vi "Initialize.vi"(8 "error in":errorcluster, 10 "parameters":variant, 11 "voltage in":refnum<class "voltage node.lvclass">) -> (0 "error out":errorcluster, 2 "summary":T2[](array[typedef]), 3 "data value reference":T1)   [LabVIEW 2013, in "voltage node.lvclass"]
doc: "This Vi initializes the data of a node its default state.\nThe object is not created inside of this ViI, beacuase it is created from a File depending on user selection."
uses:
  voltage node.lvclass
  CEF_TreeControl/Node/Summary.ctl
  CEF_TreeControl/Node/NodeRef.ctl
  CEF_TreeControl/Node/NISE_CEF_Node.lvclass
  channel configuration/ChannelData.ctl
  channel node/channel node.lvclass
  channel node/Write Channel info.vi
  channel configuration/channel configuration.lvclass
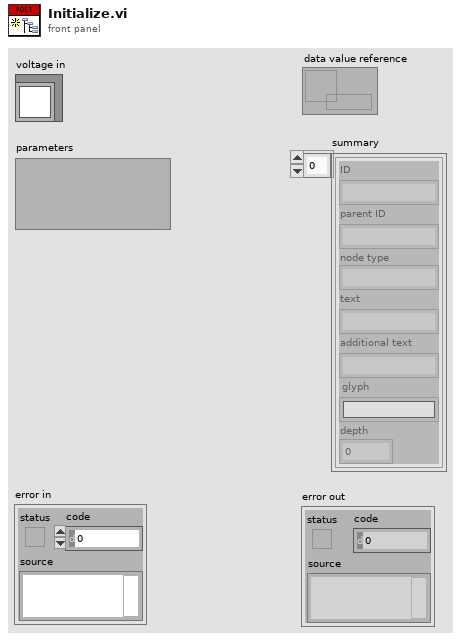
[diagram p1: front panel]
types:
  T1 = typedef "NISE_CEF_Node.lvclass/NodeRef.ctl" = refnum<data-value>
  T2 = typedef "NISE_CEF_Node.lvclass/Summary.ctl" = cluster{"ID":string, "parent ID":string, "node type":string, "text":string, "additional text":string, "glyph":string, "depth":i32}
  T3 = typedef "channel configuration.lvclass/ChannelData.ctl" = cluster{"channel group":string, "channel name":string, "IO":string, "sensor ID":string, "description":string, "system":string, "channel type":string}
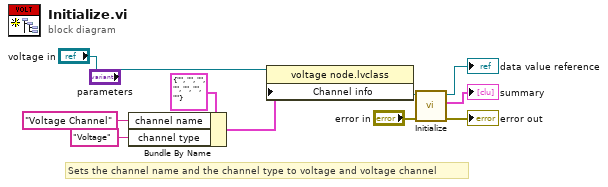
[diagram p0: block diagram]
diagram:
  # "Sets the channel name and the channel type to voltage and voltage channel"
  n1 = Bundle By Name(cluster=T3 {"channel group"="", "channel name"="", "IO"="", "sensor ID"="", "description"="", "system"="", "channel type"=""} ("channel info"), "channel name"="Voltage Channel" ("channel Name"), "channel type"="Voltage" ("channelType")) -> (w3:T3)
  n2 = property class="voltage node.lvclass"(reference="voltage in", "Channel info"=w3) -> (reference out=w5:refnum<class "voltage node.lvclass">)  [unwired: 1 in, 1 out]
  n3 = call-parent "Initialize.vi"("error in"="error in", "node in"=w5) -> ("error out"=→"error out":errorcluster, "summary"=→"summary":T2[], "data value reference"=→"data value reference":T1)  [unwired: 7 in]
